vi "read.vi"   [LabVIEW 2017]
doc: "refer：队列索引\nindex：当refer是数组时，用来选择队列的索引，当refer是单个索引时，没有作用\nwait：队列里没有信息时，是否等待，默认false\nto：消息执行器的消息处理帧名称，可以理解成消息接收者\ndata：消息携带的数据\nvaildData：wait为false的时候，vaildData为false，表示数据为无效数据\nfrom：消息执行器的消息发送帧名称，可以理解成消息发送者\nremark1，remark2：附带信息，使用者可以自己定义用处"
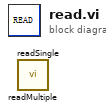
[diagram p0: block diagram]
diagram:
  n1 = call "readMultiple.vi"() -> ()  [unwired: 12 in, 8 out]
  n2 = call "readSingle.vi"() -> ()  [unwired: 12 in, 8 out]
